vi "Populate Settings Dictonary.vi"(0 "sequence file path":path, 5 "Section Name":string="Scalar", 11 "error in (no error)":errorcluster) -> (4 "setting section exists?":bool, 15 "error out":errorcluster)   [LabVIEW 2023, in "RFCalAndFixtureCharact.Common.lvlib"]
uses:
  RFCalAndFixtureCharact.Common.lvlib
  Data Cache/Settings Dictionary/Setting Keys.vi
  <vilib>/Utility/config.llb/Read Key (String).vi
  <vilib>/Utility/config.llb/NI_LVConfig.lvlib
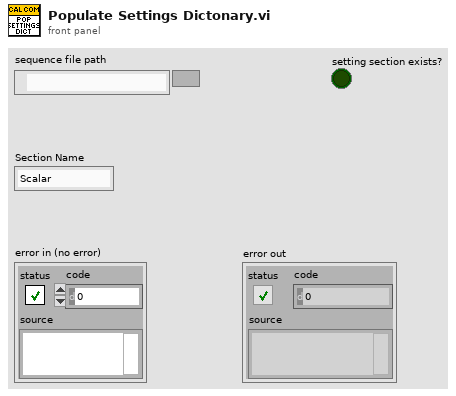
[diagram p1: front panel]
types:
  T1 = typedef "NI_LVConfig.lvlib/Config Data RefNum.ctl" = refnum<k1>
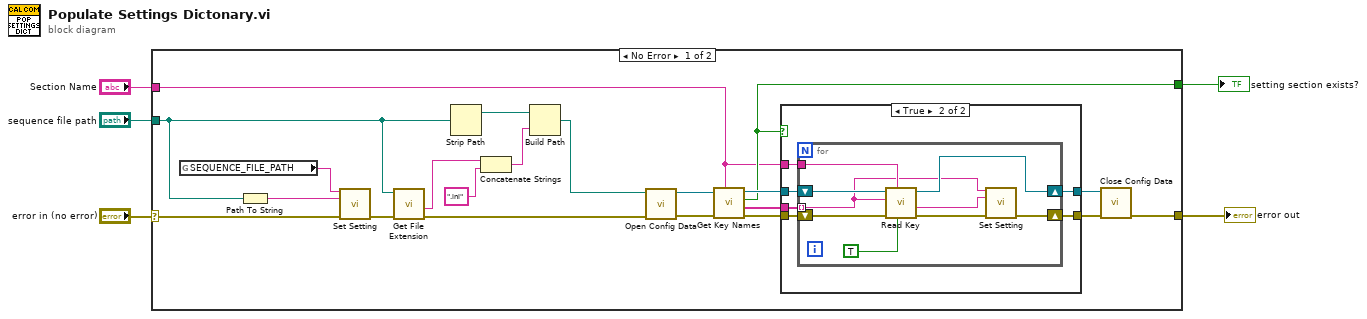
[diagram p0: block diagram]
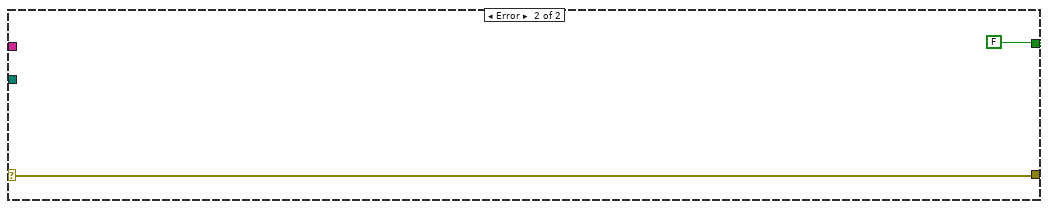
[diagram p3: hidden frame]
diagram:
  n1 = case shown="No Error" "error in (no error)" {
    selector: "error in (no error)" -> [w14 w45]
    tunnel: "sequence file path" -> [w12 _]
    tunnel: [w16 w45] -> w3
    tunnel: "Section Name" -> [w6 _]
    tunnel: [w7 FALSE] -> w1
    frame No Error {
      n2 = global read "Setting Keys.vi" "SEQUENCE_FILE_PATH"() -> (w15:string)
      n3 = Path To String(path=w12) -> (string=w11:string)
      n4 = call "Set Setting.vi"("Setting name"=w15, "Setting value"=w11, "error in (no error)"=w14) -> ("error out"=w13:errorcluster)  [unwired: 10 in, 2 out]
      n5 = call <vilib>:"Get File Extension.vi"("error in (no error)"=w13, "file"=w12) -> ("error out"=w17:errorcluster, "filename without extension"=w26:string)  [unwired: 5 in, 3 out]
      n6 = Strip Path(path=w12) -> (stripped path=w24:path)  [unwired: 1 out]
      n7 = Concatenate Strings(w26, ".ini" ("lowercase file extension")) -> (w23:string)
      n8 = Build Path(base path=w24, name or relative path=w23) -> (appended path=w22:path)
      n9 = call <vilib>:"Open Config Data.vi"("error in (no error)"=w17, "configuration file path"=w22) -> ("error out"=w20:errorcluster, "refnum"=w21:T1)  [unwired: 7 in, 1 out]
      n10 = call <vilib>:"Get Key Names.vi"("section"=w6, "error in (no error)"=w20, "refnum"=w21) -> ("error out"=w19:errorcluster, "key names"=w9:string[], "section exists?"=w7:bool, "refnum out"=w18:T1)  [unwired: 5 in]
      n11 = case shown="True" w7 {
        tunnel: w19 -> [w28 w34]
        tunnel: w18 -> [w27 w33]
        tunnel: w6 -> [_ w32]
        tunnel: [w27 w31] -> w10
        tunnel: w9 -> [_ w30]
        tunnel: [w28 w29] -> w8
        frame False {
        }
        frame True {
          n12 = for {
            tunnel: w30 -> [w36] mode=indexing
            shift-right: [w37] -> w29
            shift-left: w34 -> [w43]
            tunnel: w32 -> [w41]
            shift-right: [w39] -> w31
            shift-left: w33 -> [w42]
            n13 = call-poly <vilib>:"Read Key.vi"("read raw string? (F)"=TRUE, "section"=w41, "error in (no error)"=w43, "key"=w36, "refnum"=w42) -> ("error out"=w38:errorcluster, "value"=w35:string, "refnum out"=w39:T1)  [unwired: 3 in, 1 out]
            n14 = call "Set Setting.vi"("Setting name"=w36, "Setting value"=w35, "error in (no error)"=w38) -> ("error out"=w37:errorcluster)  [unwired: 10 in, 2 out]
          }
        }
      }
      n15 = call <vilib>:"Close Config Data.vi"("error in (no error)"=w8, "refnum"=w10) -> ("error out"=w16:errorcluster)  [unwired: 8 in, 1 out]
    }
    frame Error {
    }
  }
  "error out" <- w3
  "setting section exists?" <- w1
